vi "OpenGhostDrve.vi"(8 "error in (no error)":errorcluster) -> (0 "error out":errorcluster, 1 "RobotDriveRef":T2={"RobotDriveDevRef"={"DevStatus"={"status"=FALSE, "code"=0, "source"=""}, "Motors[]"=[], "Square Inputs"=FALSE, "Max Output"=0.0}, "Control Mode"=enum."Percent VBus", "Motor Settings"={"Wheel Radius"=0.0, "Encoder Ticks Per Rev"=0.0, "Gear Ratio"=0.0, "ClimbRev"=0.0}, "Default Control Mode"=enum."Unchanged / Invalid", "Speed Mag"=0.0, "Left Set Speed"=0.0, "Right Set Speed"=0.0}, 2 "Control Mode":T1)   [LabVIEW 2015]
uses:
  Advanced Drive VIs/RobotDrive Type Def.ctl
  <vilib>/Rock Robotics/WPI/MotorControl/WPI_MotorControlDeviceRef.ctl
  <vilib>/Rock Robotics/WPI/MotorControl/WPI_MotorControlType.ctl
  <vilib>/Rock Robotics/SystemInterfaces/DIO/FPGA_DIOPWMChannel.ctl
  <vilib>/Rock Robotics/WPI/PWM/WPI_PWMDeadband.ctl
  <vilib>/Rock Robotics/WPI/CAN/Jaguar/SubVIs/WPI_CANJaguar_ControlMode.ctl
  <vilib>/Rock Robotics/WPI/CAN/TalonSRX/WPI_CANTalonSRX_APIControlMode.ctl
  Advanced Drive VIs/Drive Motor Settings.ctl
  <vilib>/Rock Robotics/WPI/MotorControl/WPI_MotorControlOpenCANTalonSRX.vi
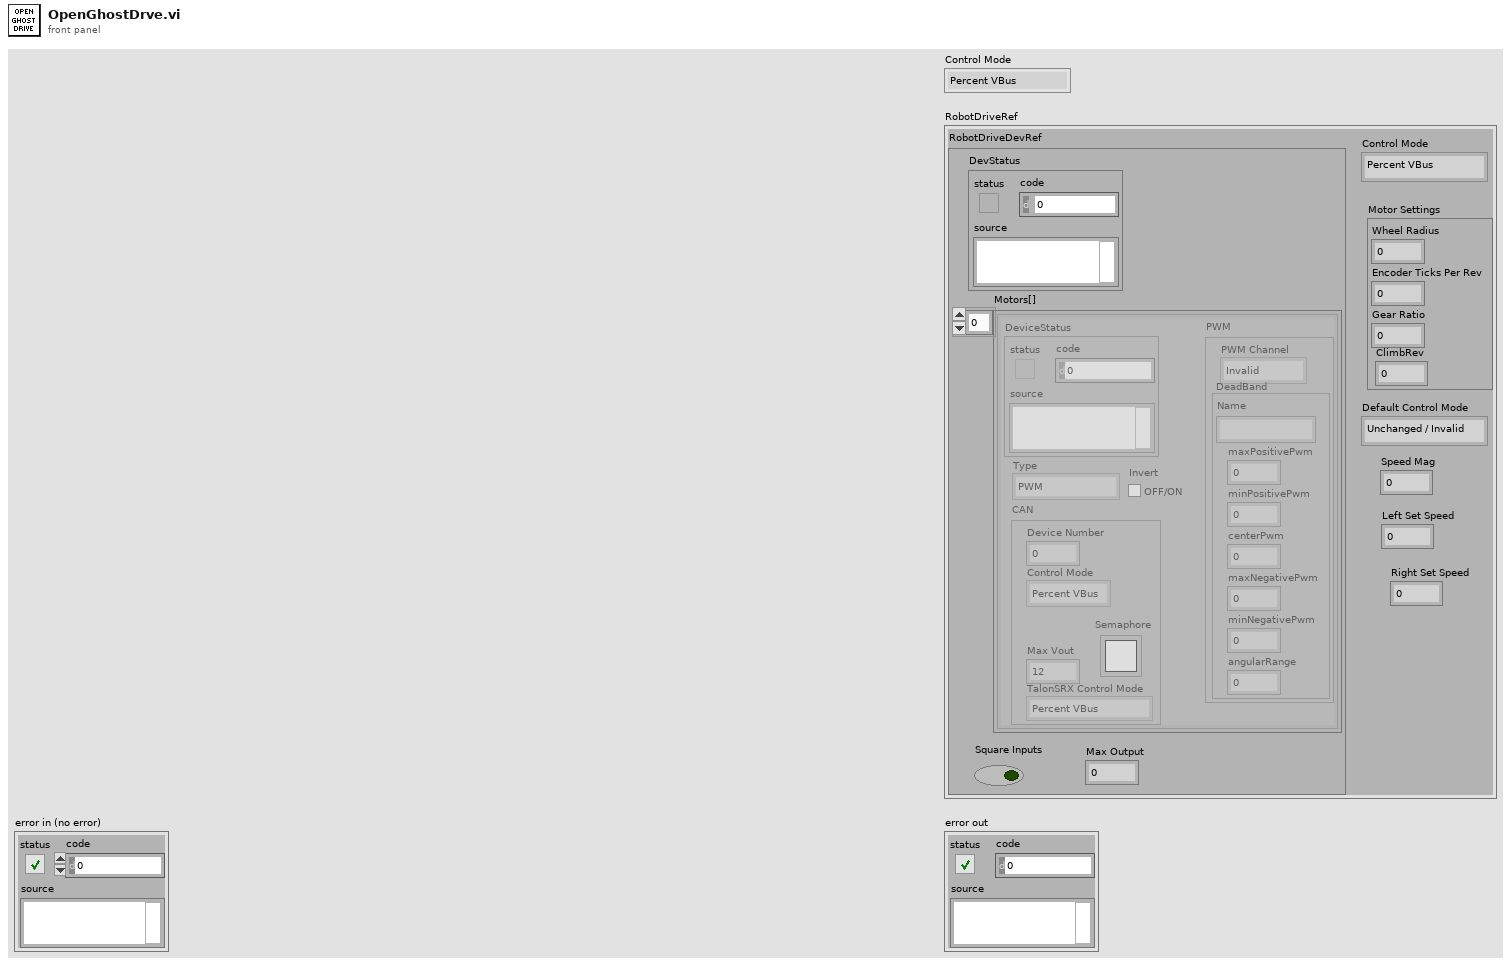
[diagram p1: front panel]
types:
  T1 = typedef "WPI_CANTalonSRX_APIControlMode.ctl" = enum8{"Percent VBus", "Speed", "Position", "Slave", "Unchanged / Invalid", "Voltage Compensation", "Current", "Motion Profile"}
  T2 = typedef "RobotDrive Type Def.ctl" = cluster{"RobotDriveDevRef":cluster{"DevStatus":errorcluster, "Motors[]":T3[], "Square Inputs":bool, "Max Output":dbl}, "Control Mode":T1, "Motor Settings":T9, "Default Control Mode":T1, "Speed Mag":dbl, "Left Set Speed":dbl, "Right Set Speed":dbl}
  T3 = typedef "WPI_MotorControlDeviceRef.ctl" = cluster{"DeviceStatus":errorcluster, "Type":T4, "PWM":cluster{"PWM Channel":T5, "DeadBand":T6}, "CAN":cluster{"Device Number":u8, "Control Mode":T7, "Semaphore":T8, "Max Vout":dbl, "TalonSRX Control Mode":T1}, "Invert":bool}
  T4 = typedef "WPI_MotorControlType.ctl" = enum16{"PWM", "CAN", "CANTalonSRX"}
  T5 = typedef "FPGA_DIOPWMChannel.ctl" = enum8{"PWM 0", "PWM 1", "PWM 2", "PWM 3", "PWM 4", "PWM 5", "PWM 6", "PWM 7", "PWM 8", "PWM 9", "PWM MXP 0", "PWM MXP 1", "PWM MXP 2", "PWM MXP 3", "PWM MXP 4", "PWM MXP 5", "PWM MXP 6", "PWM MXP 7", "PWM MXP 8", "PWM MXP 9", "Invalid"}
  T6 = typedef "WPI_PWMDeadband.ctl" = cluster{"Name":string, "maxPositivePwm":i32, "minPositivePwm":i32, "centerPwm":i32, "maxNegativePwm":i32, "minNegativePwm":i32, "angularRange":u16}
  T7 = typedef "WPI_CANJaguar_ControlMode.ctl" = enum8{"Percent VBus", "Current", "Speed", "Position", "Voltage"}
  T8 = typedef "Semaphore RefNum" = refnum<k1>
  T9 = typedef "Drive Motor Settings.ctl" = cluster{"Wheel Radius":dbl, "Encoder Ticks Per Rev":dbl, "Gear Ratio":dbl, "ClimbRev":dbl}
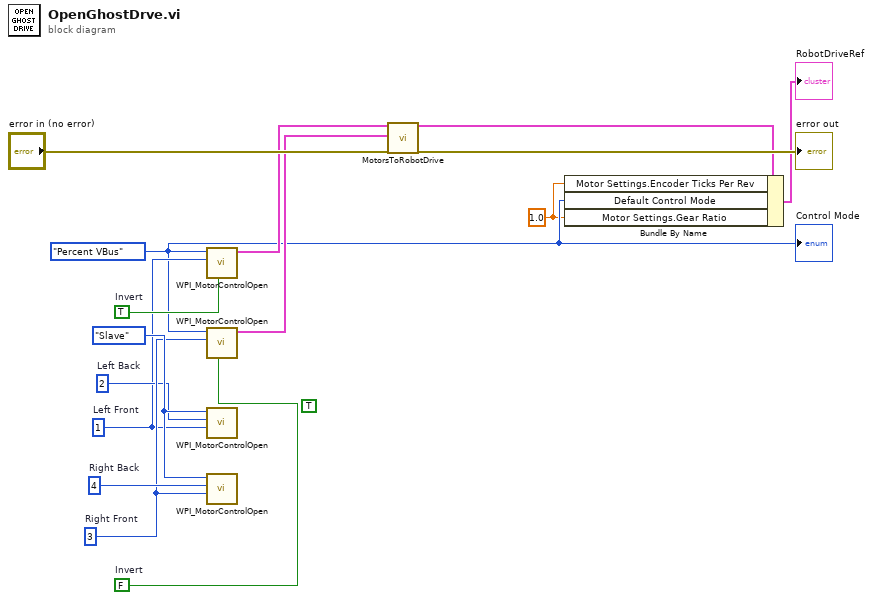
[diagram p0: block diagram]
diagram:
  w1 = 1.0 ("Motor Settings.Encoder Ticks Per Rev")
  (unwired) TRUE
  w12 = TRUE  # Invert
  w11 = FALSE  # Invert
  w8 = u8 4  # Right Back
  w7 = u8 3  # Right Front
  w15 = WPI_CANTalonSRX_APIControlMode."Slave" ("Control Mode")
  w6 = u8 2  # Left Back
  w5 = u8 1  # Left Front
  w2 = WPI_CANTalonSRX_APIControlMode."Percent VBus" ("Control Mode")
  n1 = call-poly <vilib>:"WPI_MotorControlOpen.vi"("Invert"=w12, "Device Number"=w5, "Control Mode"=w2) -> ("MotorControlDeviceRef"=w9:T3)  [unwired: 7 in, 1 out]
  n2 = call-poly <vilib>:"WPI_MotorControlOpen.vi"("Invert"=w11, "Device Number"=w7, "Control Mode"=w2) -> ("MotorControlDeviceRef"=w10:T3)  [unwired: 7 in, 1 out]
  n3 = call-poly <vilib>:"WPI_MotorControlOpen.vi"("Master Device Number"=w5, "Device Number"=w6, "Control Mode"=w15) -> ()  [unwired: 7 in, 2 out]
  n4 = call-poly <vilib>:"WPI_MotorControlOpen.vi"("Master Device Number"=w7, "Device Number"=w8, "Control Mode"=w15) -> ()  [unwired: 7 in, 2 out]
  n5 = call "MotorsToRobotDrive.vi"("Left"=w9, "Right"=w10, "error in"="error in (no error)") -> ("RobotDriveRef"=w4:T2, "error out"=→"error out":errorcluster)  [unwired: 15 in]
  n6 = Bundle By Name(cluster=w4, "Motor Settings.Encoder Ticks Per Rev"=w1, "Default Control Mode"=w2, "Motor Settings.Gear Ratio"=w1) -> (→"RobotDriveRef":T2)
  "Control Mode" <- w2
